vi "rpm.vi"(4 "error in":errorcluster, 7 "RPM configuration":string="{\n  \"type\": \"RPM\",\n  \"listen_port\": 8600,\n  \"location\": {\n    \"x\": 0,\n    \"y\": 0,\n    \"z\": 0\n  },\n  \"rotation\": {\n    \"pitch\": 0,\n    \"yaw\": 0,\n    \"roll\": 0\n  },\n  \"wheelNumber\": 3\n}") -> (0 "error out":errorcluster, 1 "RPM configuration":string, 2 "Raw data":string, 3 "RPM Sample":cluster{"wheel_number":i32, "wheel_RPM":sgl})   [LabVIEW 2019]
doc: "Configure and read the RPM information of the vehicle."
uses:
  controls/Header.ctl
  tools/simx_common.vi
panel:
  out "Header":T1 {"game_time" format="%#_10g"}
  in  "data format":T2
  in  "rpm_connection":refnum<k5>
  in  "null connection":refnum<k5>
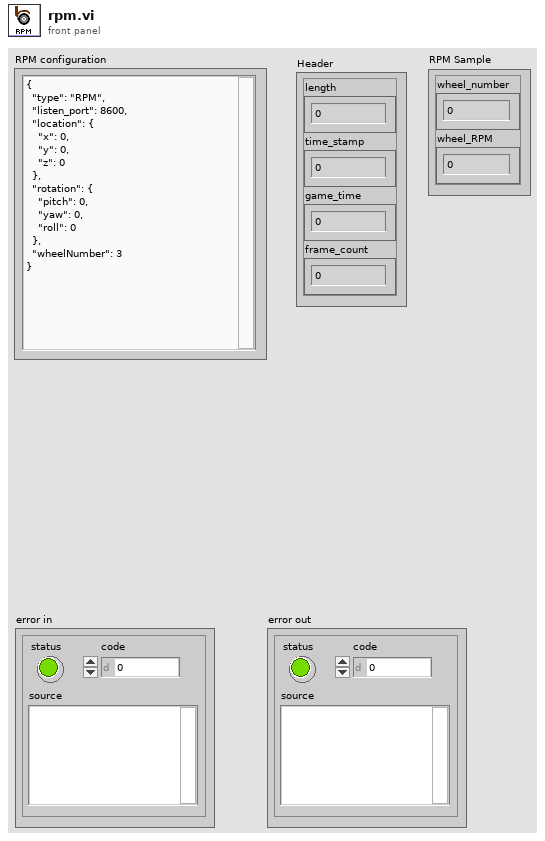
[diagram p1: front panel]
types:
  T1 = typedef "Header.ctl" = cluster{"length":u32, "time_stamp":u32, "game_time":sgl, "frame_count":u32}
  T2 = cluster{"wheel_number":i32, "wheel_speed_lf":sgl}
  T3 = typedef "simx_connection.ctl" = cluster{"Config":T4, "Connections":T7, "Map":cluster{"lanes":cluster{"x":dbl[], "y":dbl[], "z":dbl[]}, "StartPosition":cluster{"start_points":T8, "StartRotation":dbl[], "StartLocation":dbl[]}, "Draw Map Size":T9, "DrawArea":cluster{"min_Y":dbl, "min_X":dbl, "Scale X":dbl, "Scale Y":dbl}, "Map":picture, "Map Geojson":string}}
  T4 = typedef "config.ctl" = cluster{"Trajectory":T5, "Weather":T6}
  T5 = typedef "trajectory.ctl" = cluster{"Number of frames":i32, "Frame number":i32, "Trajectory":string}
  T6 = typedef "weather.ctl" = cluster{"id":string}
  T7 = typedef "connections.ctl" = cluster{"Simulator Connection":refnum<k5>, "server_ip":string, "Port":i32, "Sensor connections":refnum<k5>[]}
  T8 = typedef "start_points.ctl" = cluster{"locations":dbl[][], "rotations":dbl[][], "type":string[]}
  T9 = typedef "LVBoundsTypeDef.ctl" = cluster{"Width":u32, "Height":u32}
  T10 = enum16{"big-endian, network order", "native, host order", "little-endian"}
  T11 = typedef "sensor_sample.ctl" = cluster{"Header":T1, "data out":string}
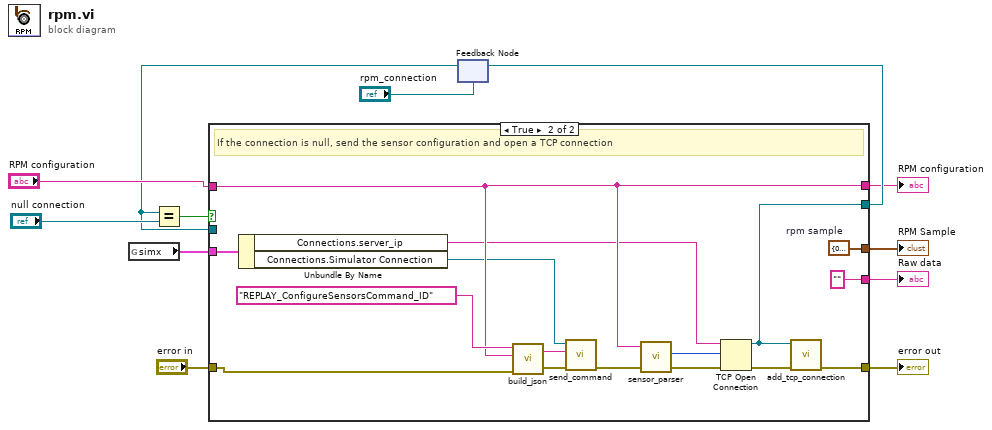
[diagram p0: block diagram]
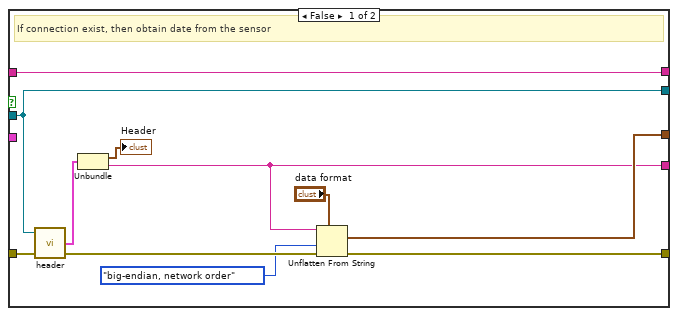
[diagram p2: hidden frame]
diagram:
  n1 = global read "simx_common.vi" "simx"() -> (w1:T3)
  n2 = feedback #1("rpm_connection") -> (w7:refnum<k5>)
  n3 = Equal?(x=w7, y="null connection") -> (x = y?=w9:bool)
  n4 = case shown="True" w9 {
    tunnel: [w19 w27] -> w4
    tunnel: "RPM configuration" -> [w15 w29]
    tunnel: [w18 w26] -> w10
    tunnel: w7 -> [w18 _]
    tunnel: "error in" -> [w20 w33]
    tunnel: [w17 w34] -> w5
    tunnel: [w15 w29] -> w3
    tunnel: [w14 "" ("data out")] -> w2
    tunnel: w1 -> [_ w31]
    frame False {
      # "If connection exist, then obtain date from the sensor"
      n5 = call "header.vi"("error in"=w20, "TCP Network Connection in"=w18) -> ("error out"=w22:errorcluster, "Sensor sample"=w23:T11)  [unwired: 1 in, 1 out]
      n6 = Unbundle(w23) -> ("Header"=→"Header":T1, "data out"=w14:string)
      n7 = Unflatten From String(type="data format", binary string=w14, byte order (0:big-endian, network order)=T10."big-endian, network order", error in (no error)=w22) -> (value=w17:T2, error out=w19:errorcluster)  [unwired: 1 in, 1 out]
    }
    frame True {
      w34 = T2 {"wheel_number"=0, "wheel_speed_lf"=0.0}  # rpm sample
      # "If the connection is null, send the sensor configuration and open a TCP connection"
      n8 = Unbundle By Name(w31) -> ("Connections.server_ip"=w24:string, "Connections.Simulator Connection"=w25:refnum<k5>)
      n9 = call "build_json.vi"("error in"=w33, "Message"=w29, "Command_ID"="REPLAY_ConfigureSensorsCommand_ID") -> ("error out"=w37:errorcluster, "JSON Out"=w38:string)  [unwired: 1 in]
      n10 = call "send_command.vi"("error in"=w37, "JSON Command"=w38, "TCP Network Connection in"=w25) -> ("error out"=w36:errorcluster)  [unwired: 1 in, 3 out]
      n11 = call "sensor_parser.vi"("Sensor configuration"=w29, "error in"=w36) -> ("Port out"=w28:u16, "error out"=w30:errorcluster)  [unwired: 1 in, 2 out]
      n12 = TCP Open Connection(address=w24, remote port or service name=w28, error in (no error)=w30) -> (connection ID=w26:refnum<k5>, error out=w35:errorcluster)  [unwired: 2 in]
      n13 = call "add_tcp_connection.vi"("error in"=w35, "Sensor connection"=w26) -> ("error out"=w27:errorcluster)  [unwired: 5 in]
    }
  }
  "RPM Sample" <- w5
  "error out" <- w4
  "RPM configuration" <- w3
  "Raw data" <- w2
  n14 = feedback-in #1(w10) -> ()
